vi "parse - find tokens.vi"(4 "tokens wanted":string[](array[string])=["Time", "SRS_Vx\\s*\\(V\\)", "Keith_Volts", "LTC\\s*CH2"], 6 "all tokens":string[](array[string])=["Time", "SRS_Vx\\s*\\(V\\)", "Keith_Volts", "LTC\\s*CH2", "SRS_Vy\\s*\\(V\\)", "ITC\\s*CH1", "ITC\\s*CH2"], 11 "line":string="Time\tSRS_Vx (V)\tSRS_Vy (V)\tLTC CH2\tKeith_Volts\tITC CH1\tITC CH2") -> (2 "token indices":i32[](array[numeric])=[0, 1, 3, 2])   [LabVIEW 2012]
panel:
  out "token list":string="(Time|SRS_Vx\\s*\\(V\\)|Keith_Volts|LTC\\s*CH2|Keith_Volts|ITC\\s*CH1|ITC\\s*CH2)\\s*\\r?"
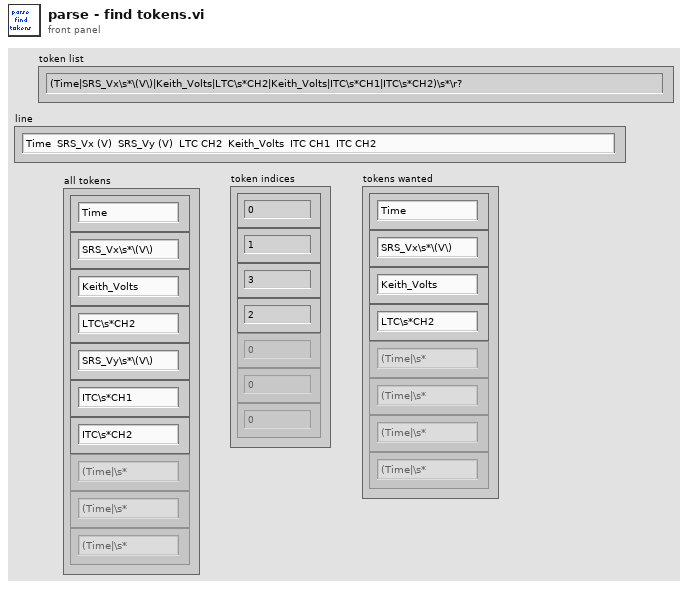
[diagram p1: front panel]
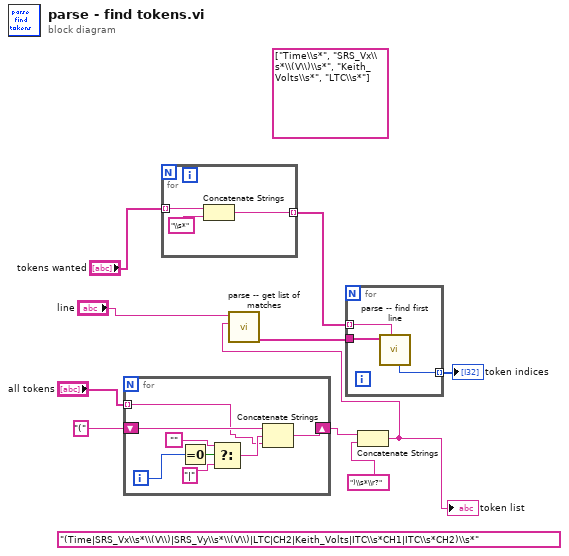
[diagram p0: block diagram]
diagram:
  (unwired) string[] ["Time\\s*", "SRS_Vx\\s*\\(V\\)\\s*", "Keith_Volts\\s*", "LTC\\s*"]
  (unwired) "(Time|SRS_Vx\\s*\\(V\\)|SRS_Vy\\s*\\(V\\)|LTC|CH2|Keith_Volts|ITC\\s*CH1|ITC\\s*CH2)\\s*" ("regexp")
  n1 = for {
    tunnel: "all tokens" -> [w11] mode=indexing
    shift-right: [w17] -> w5
    shift-left: "(" ("regexp") -> [w18]
    i -> [w16]
    n2 = Equal To 0?(x=w16) -> (x = 0?=w15:bool)
    n3 = Select(t="", s=w15, f="|" ("regexp")) -> (s? t:f=w12:string)
    n4 = Concatenate Strings(w18, w12, w11) -> (w17:string)
  }
  n5 = for {
    tunnel: "tokens wanted" -> [w21] mode=indexing
    tunnel: [w19] -> w1 mode=indexing
    n6 = Concatenate Strings(w21, "\\s*" ("regexp")) -> (w19:string)
  }
  n7 = Concatenate Strings(w5, ")\\s*\\r?" ("regexp")) -> (w3:string)
  "token list" <- w3
  n8 = call "parse -- get list of matches.vi"("regexp"=w3, "string"="line") -> ("Array"=w10:string[])  [unwired: 7 in, 2 out]
  n9 = for {
    tunnel: w10 -> [w24]
    tunnel: w1 -> [w23] mode=indexing
    tunnel: [w22] -> w9 mode=indexing
    n10 = call "parse -- find first line.vi"("regexp"=w23, "string array"=w24) -> ("index"=w22:i32)  [unwired: 5 in, 4 out]
  }
  "token indices" <- w9
